vi "oval_results.vi"(10 "Solution":dbl[](array[numeric]), 11 "ovalization_data":T1={"AngOval"=[0.0, 60.0, 120.0, 22.5, 45.0, 67.5, 90.0, 112.5, 135.0, 157.5, 180.0], "OvalDiam"=[324.25, 324.6, 324.55, 324.25, 324.55, 324.65, 324.6, 324.65, 324.55, 324.5, 324.4], "Plots"={"Ref"={"X"=[], "Y"=[]}, "Elipse"={"X"=[], "Y"=[]}, "Points"={"X"=[], "Y"=[]}}, "Ampliation"=100.0, "Results"={"MD"=0.0, "mD"=0.0, "Dmed"=0.0, "Oval"=0.0, "ang"=0.0, "X0"=0.0, "Y0"=0.0}}) -> (3 "output ovalization_data-out":T1={"AngOval"=[0.0, 60.0, 120.0, 22.5, 45.0, 67.5, 90.0, 112.5, 135.0, 157.5, 180.0], "OvalDiam"=[324.25, 324.6, 324.55, 324.25, 324.55, 324.65, 324.6, 324.65, 324.55, 324.5, 324.4], "Plots"={"Ref"={"X"=[], "Y"=[]}, "Elipse"={"X"=[], "Y"=[]}, "Points"={"X"=[], "Y"=[]}}, "Ampliation"=100.0, "Results"={"MD"=0.0, "mD"=0.0, "Dmed"=0.0, "Oval"=0.0, "ang"=0.0, "X0"=0.0, "Y0"=0.0}})   [LabVIEW 2016]
uses:
  ovalization_data.ctl
  <vilib>/Analysis/baseanly.llb/Mean (DBL).vi
  <vilib>/Analysis/NI_AALBase.lvlib
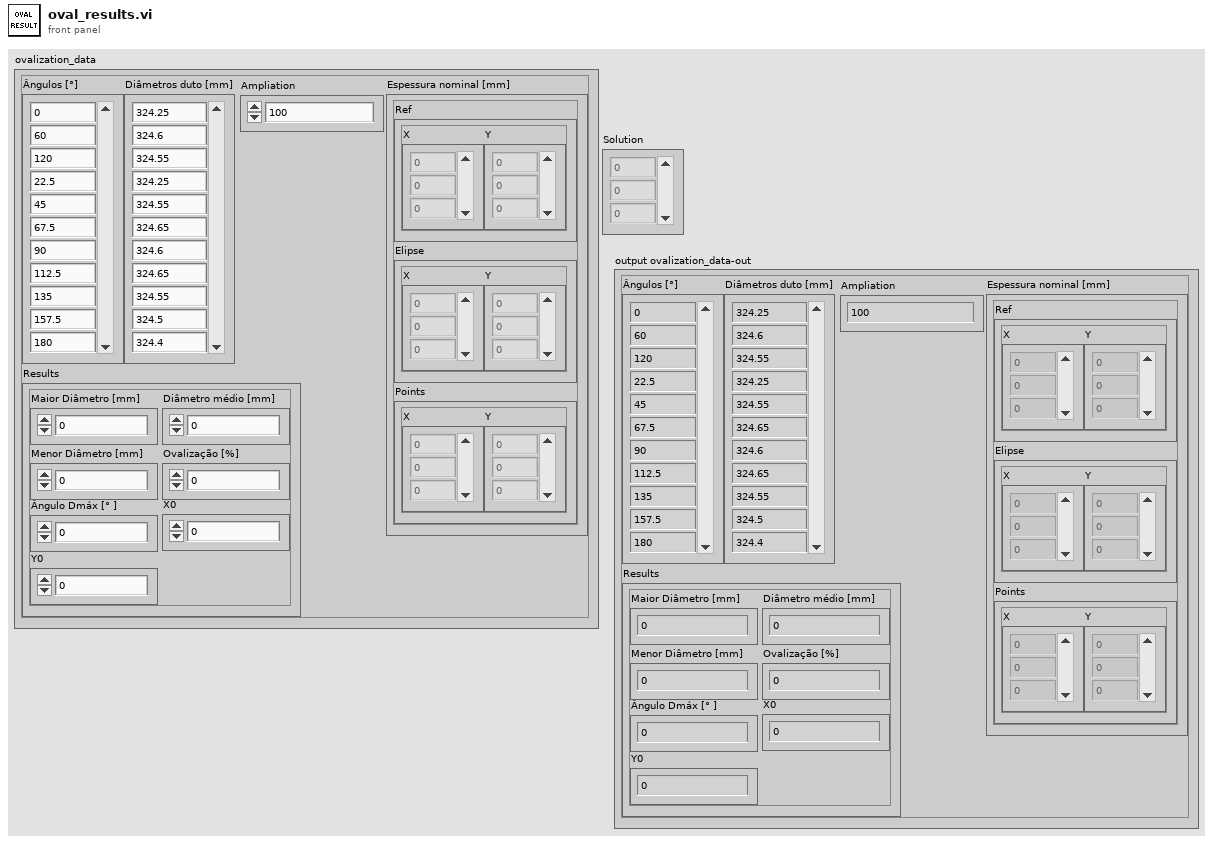
[diagram p1: front panel]
types:
  T1 = typedef "ovalization_data.ctl" = cluster{"AngOval":dbl[], "OvalDiam":dbl[], "Plots":cluster{"Ref":cluster{"X":dbl[], "Y":dbl[]}, "Elipse":cluster{"X":dbl[], "Y":dbl[]}, "Points":cluster{"X":dbl[], "Y":dbl[]}}, "Ampliation":dbl, "Results":cluster{"MD":dbl, "mD":dbl, "Dmed":dbl, "Oval":dbl, "ang":dbl, "X0":dbl, "Y0":dbl}}
  T2 = cluster{"MD":dbl, "mD":dbl, "Dmed":dbl, "Oval":dbl, "ang":dbl, "X0":dbl, "Y0":dbl}
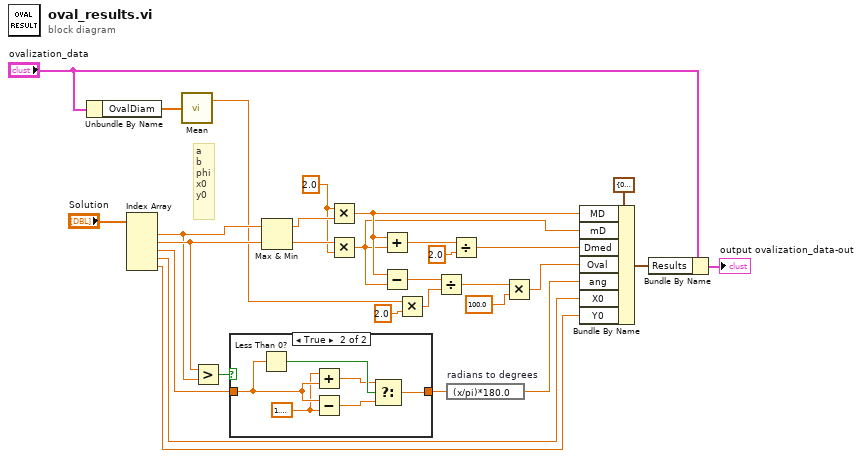
[diagram p0: block diagram]
diagram:
  w4 = 2.0 ("y")
  # "a\nb\nphi\nx0\ny0"
  n1 = Unbundle By Name("ovalization_data") -> ("OvalDiam"=w2:dbl[])
  n2 = Index Array(array="Solution") -> (element #1=w12:dbl, element #2=w13:dbl, element #3=w10:dbl, element #4=w15:dbl, element #5=w14:dbl)  [unwired: 5 in]
  n3 = call-poly <vilib>:"Mean.vi"("X"=w2) -> ("mean"=w1:dbl)  [unwired: 1 out]
  n4 = Greater?(x=w13, y=w12) -> (0:w11:bool)
  n5 = case shown="True" w11 {
    tunnel: w10 -> [w30 w35]
    tunnel: [w30 w31] -> w9
    frame False {
    }
    frame True {
      w34 = 1.5707963267948966
      n6 = Less Than 0?(x=w35) -> (x < 0?=w36:bool)
      n7 = Add(x=w34, y=w35) -> (x+y=w33:dbl)
      n8 = Subtract(x=w35, y=w34) -> (x-y=w32:dbl)
      n9 = Select(t=w33, s=w36, f=w32) -> (s? t:f=w31:dbl)
    }
  }
  n10 = Max & Min(x=w12, y=w13) -> (max(x,y)=w17:dbl, min(x,y)=w16:dbl)
  n11 = Multiply(x=w4, y=w17) -> (x*y=w26:dbl)
  n12 = Multiply(x=w16, y=w4) -> (x*y=w25:dbl)
  n13 = Add(x=w26, y=w25) -> (x+y=w29:dbl)
  n14 = Subtract(x=w26, y=w25) -> (x-y=w23:dbl)
  n15 = Multiply(x=w1, y=2.0) -> (x*y=w22:dbl)
  n16 = Divide(x=w23, y=w22) -> (x/y=w21:dbl)
  n17 = expression code="(x/pi)*180.0" "radians to degrees"(w9) -> (w18:dbl)
  n18 = Divide(x=w29, y=2.0) -> (x/y=w27:dbl)
  n19 = Multiply(x=w21, y=100.0) -> (x*y=w19:dbl)
  n20 = Bundle By Name(cluster=T2 {"MD"=0.0, "mD"=0.0, "Dmed"=0.0, "Oval"=0.0, "ang"=0.0, "X0"=0.0, "Y0"=0.0} ("Results"), "MD"=w26, "mD"=w25, "Dmed"=w27, "Oval"=w19, "ang"=w18, "X0"=w15, "Y0"=w14) -> (w6:T2)
  n21 = Bundle By Name(cluster="ovalization_data", "Results"=w6) -> (→"output ovalization_data-out":T1)
